vi "robot rocky222.vi"() -> ()   [LabVIEW 2021]
uses:
  <vilib>/userDefined/High Color/IMAQdx.ctl
  <vilib>/MakerHub/LINX/Private/Device/Type Defs/TCP Config.ctl
  <vilib>/vision/driver/NI_Vision_Acquisition_Software.lvlib
  <vilib>/vision/NI_Vision_Development_Module.lvlib
  <vilib>/MakerHub/LINX/LMH-LINX.lvlib
  <vilib>/MakerHub/LINX/Public/Peripherals/PWM/PWM Set Duty Cycle 1 Chan.vi
  <vilib>/MakerHub/LINX/Public/Utilities/Open TCP.vi
  <vilib>/MakerHub/LINX/Public/Peripherals/Digital/Digital Write N Chans.vi
  <vilib>/MakerHub/LINX/Private/Device/Device.lvlib
panel:
  in  "address ip":string
  in  "avance":bool
  in  "reculer":bool
  in  "Gauche":bool
  in  "droite":bool
  in  "Process Stop Button":bool
  in  "Stop":bool
  out "Image Out":T1(plugin-control)
  in  "TCP Configuration":T2
  in  "Duty Cycle (0-1)":dbl(slide) min=0.0 max=1.0 step=0.0005 scale=0.0..1.0
  in  "Motor Direction":bool[](array[boolean])
  in  "STOP":bool
  in  "Session In":T3
  in  "?":bool
  out "Acquired Frames per Second":dbl(knob) scale=0.0..100.0
  out "real time tracking":T1(plugin-control)
  in  "Color Plane":i32(ring)=1 items=["Red", "Green", "Blue", "Hue", "Saturation", "Luminance", "Value", "Intensity"]
  in  "MANUEL":bool
  in  "mode1":bool
  # "robot rocky"
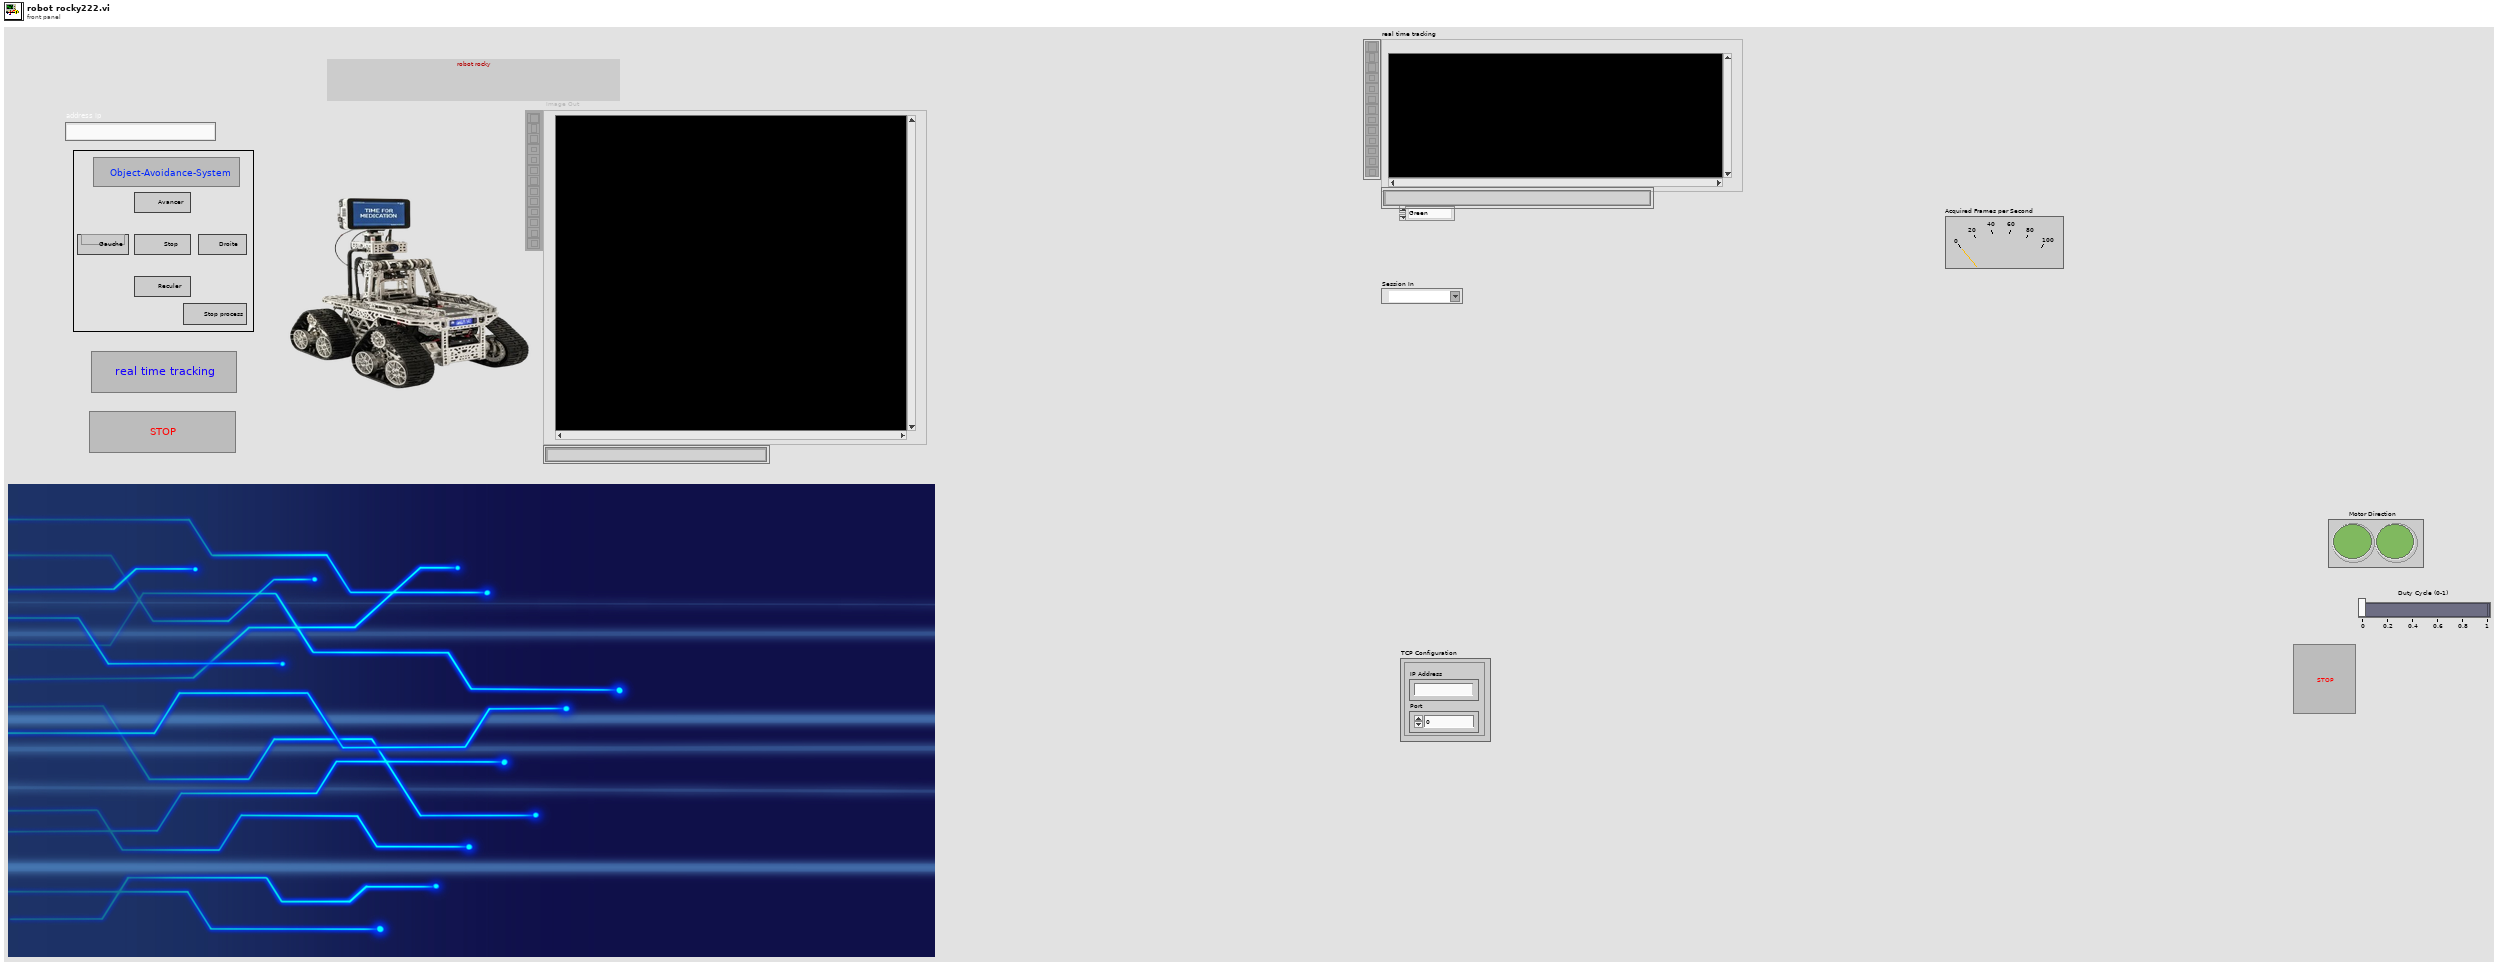
[diagram p1: front panel]
types:
  T1 = typedef "IMAQ Image.ctl" = refnum<image>
  T2 = typedef "LMH-LINX.lvlib/Device.lvlib/TCP Config.ctl" = cluster{"IP Address":string, "Port":u16}
  T3 = typedef "IMAQdx.ctl" = refnum<k21>
  T4 = typedef "Image Type" = u32
  T5 = typedef "LMH-LINX.lvlib/LINX Ref.ctl" = cluster{"IO":T6, "Interface":T7, "LINX Device Config":T8}
  T6 = typedef "LMH-LINX.lvlib/Platform.ctl" = enum16{"Remote", "Local"}
  T7 = typedef "LMH-LINX.lvlib/Interface.ctl" = enum16{"Serial", "TCP"}
  T8 = typedef "LMH-LINX.lvlib/Device.lvlib/LINX Device Config.ctl" = cluster{"Interface":T7, "COM Port":refnum<visa-resource-name>, "TCP Configuration":T2, "Device Family":u8, "Device ID":u8, "Device Name":string, "TCP Ref":refnum<k5>, "Channels":T9}
  T9 = typedef "LMH-LINX.lvlib/Channels.ctl" = cluster{"DI":u8[], "DO":u8[], "AI":u8[], "AO":u8[], "PWM":u8[], "QE":u8[], "UART":u8[], "I2C 2":u8[], "SPI":u8[], "CAN":u8[], "Servo":u8[], "AI Ref (V)":dbl, "AI Resolution (Bits)":u8, "AO Ref (V)":dbl, "AO Resolution (Bits)":u8}
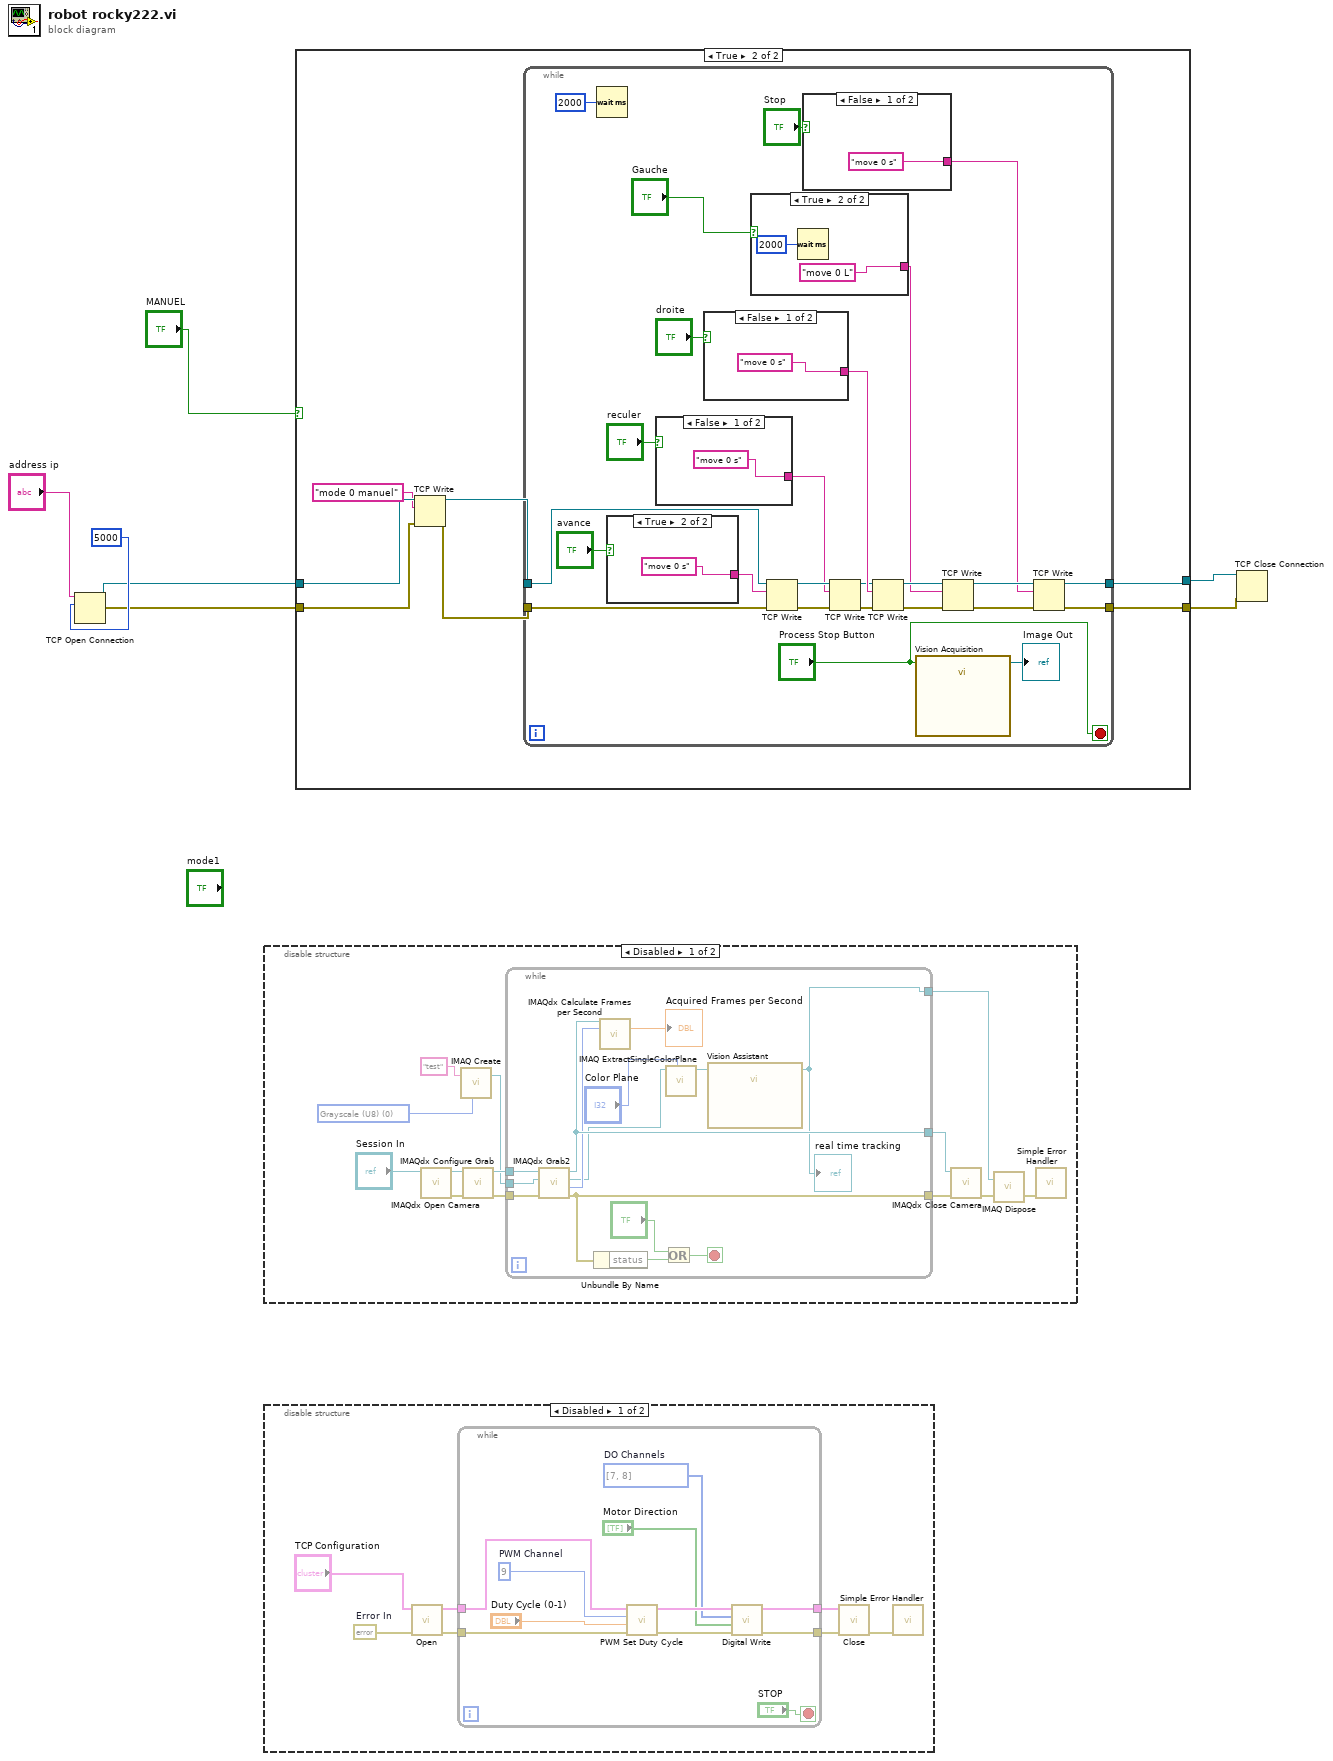
[diagram p0: block diagram]
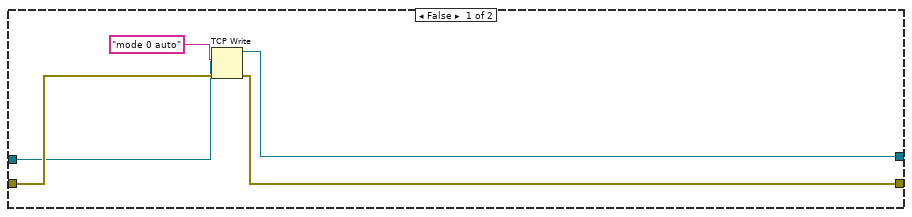
[diagram p2: hidden frame]
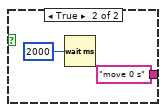
[diagram p3: hidden frame]
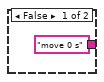
[diagram p4: hidden frame]
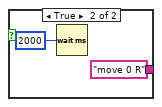
[diagram p5: hidden frame]
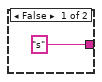
[diagram p6: hidden frame]
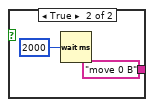
[diagram p7: hidden frame]
diagram:
  n1 = TCP Open Connection(address="address ip", remote port or service name=u16 5000) -> (connection ID=w5:refnum<k5>, error out=w4:errorcluster)  [unwired: 3 in]
  n2 = disable-structure shown="Disabled" {
    frame Disabled {
      w9 = T4 0 items=["Grayscale (U8)", "Grayscale (I16)", "Grayscale (SGL)", "Complex (CSG)", "RGB (U32)", "HSL (U32)", "RGB (U64)", "Grayscale (U16)"] ("Image Type")
      n3 = call <vilib>:"IMAQdx Open Camera.vi"("Session In"="Session In") -> ("error out"=w18:errorcluster, "Session Out"=w19:T3)  [unwired: 9 in]
      n4 = call "IMAQ Create"("Image Name"="test", "Image Type"=w9) -> ("New Image"=w8:T1)  [unwired: 3 in, 1 out]
      n5 = call <vilib>:"IMAQdx Configure Grab.vi"("error in"=w18, "Session In"=w19) -> ("error out"=w16:errorcluster, "Session Out"=w17:T3)  [unwired: 8 in]
      n6 = while {
        tunnel: w17 -> [w34]
        tunnel: w16 -> [w33]
        tunnel: [w26] -> w15
        tunnel: [w30] -> w14
        tunnel: [w21] -> w13
        tunnel: w8 -> [w28]
        stop <- w32 stop-if-true
        n7 = call <vilib>:"IMAQdx Grab2.vi"("error in"=w33, "Image In"=w28, "Session In"=w34) -> ("error out"=w30:errorcluster, "Buffer Number Out"=w25:u32, "Image Out"=w24:T1, "Session Out"=w26:T3)  [unwired: 5 in]
        n8 = Unbundle By Name(w30) -> ("status"=w29:bool)
        n9 = call <vilib>:"IMAQdx Calculate Frames per Second.vi"("Session In"=w26, "Buffer Number"=w25) -> ("Acquired Frames per Second"=→"Acquired Frames per Second":dbl)  [unwired: 7 in, 6 out]
        n10 = Or(x="?", y=w29) -> (x .or. y?=w32:bool)
        n11 = call "IMAQ ExtractSingleColorPlane"("Color Plane"="Color Plane", "Image Src"=w24) -> ("Image Dst Out"=w22:T1)  [unwired: 8 in, 1 out]
        n12 = call "Vision Assistant"("Image In"=w22) -> ("Image Out"=w21:T1)  [unwired: 25 in, 1 out]
        "real time tracking" <- w21
      }
      n13 = call <vilib>:"IMAQdx Close Camera.vi"("error in"=w14, "Session In"=w15) -> ("error out"=w12:errorcluster)  [unwired: 9 in]
      n14 = call "IMAQ Dispose"("Image"=w13, "error in (no error)"=w12) -> ("error out"=w11:errorcluster)  [unwired: 4 in]
      n15 = call <vilib>:"Simple Error Handler.vi"("error in (no error)"=w11) -> ()  [unwired: 4 in, 5 out]
    }
    frame Enabled {
    }
  }
  n16 = disable-structure shown="Disabled" {
    frame Disabled {
      w39 = errorcluster {"status"=FALSE, "code"=0, "source"=""}  # Error In
      n17 = call-poly <vilib>:"Open.vi"("Error In"=w39, "TCP Configuration"="TCP Configuration") -> ("Error Out"=w40:errorcluster, "LINX Resource"=w41:T5)  [unwired: 7 in, 1 out]
      n18 = while {
        tunnel: w41 -> [w52]
        tunnel: w40 -> [w51]
        tunnel: [w46] -> w37
        tunnel: [w45] -> w38
        stop <- "STOP" stop-if-true
        w50 = u8 9  # PWM Channel
        w42 = u8[] [7, 8]  # DO Channels
        n19 = call-poly <vilib>:"PWM Set Duty Cycle.vi"("Error In"=w51, "Duty Cycle (0-1)"="Duty Cycle (0-1)", "PWM Channel"=w50, "LINX Resource"=w52) -> ("Error Out"=w47:errorcluster, "LINX Resource"=w48:T5)  [unwired: 6 in]
        n20 = call-poly <vilib>:"Digital Write.vi"("Error In"=w47, "Values"="Motor Direction", "DO Channels"=w42, "LINX Resource"=w48) -> ("Error Out"=w46:errorcluster, "LINX Resource"=w45:T5)  [unwired: 6 in]
      }
      n21 = call <vilib>:"Close.vi"("Error In"=w37, "LINX Resource"=w38) -> ("Error Out"=w36:errorcluster)  [unwired: 9 in]
      n22 = call <vilib>:"Simple Error Handler.vi"("error in (no error)"=w36) -> ()  [unwired: 4 in, 5 out]
    }
    frame Enabled {
    }
  }
  n23 = case shown="True" "MANUEL" {
    tunnel: w5 -> [w55 w62]
    tunnel: w4 -> [w56 w59]
    tunnel: [w54 w64] -> w3
    tunnel: [w53 w63] -> w2
    frame False {
      n24 = TCP Write(connection ID=w55, data in="mode 0 auto", error in (no error)=w56) -> (connection ID out=w54:refnum<k5>, error out=w53:errorcluster)  [unwired: 1 in, 1 out]
    }
    frame True {
      n25 = TCP Write(connection ID=w62, data in="mode 0 manuel", error in (no error)=w59) -> (connection ID out=w60:refnum<k5>, error out=w58:errorcluster)  [unwired: 1 in, 1 out]
      n26 = while {
        tunnel: w60 -> [w89]
        tunnel: w58 -> [w88]
        tunnel: [w72] -> w64
        tunnel: [w71] -> w63
        stop <- "Process Stop Button" stop-if-true
        n27 = Wait (ms)(milliseconds to wait=u32 2000) -> ()  [unwired: 1 out]
        n28 = case shown="True" "avance" {
          tunnel: ["s" "move 0 s"] -> w85
          frame False {
          }
          frame True {
          }
        }
        n29 = case shown="False" "reculer" {
          tunnel: ["move 0 s" "move 0 B"] -> w84
          frame False {
          }
          frame True {
            n30 = Wait (ms)(milliseconds to wait=u32 2000) -> ()  [unwired: 1 out]
          }
        }
        n31 = case shown="False" "droite" {
          tunnel: ["move 0 s" "move 0 R"] -> w83
          frame False {
          }
          frame True {
            n32 = Wait (ms)(milliseconds to wait=u32 2000) -> ()  [unwired: 1 out]
          }
        }
        n33 = case shown="True" "Gauche" {
          tunnel: ["move 0 s" "move 0 L"] -> w78
          frame False {
          }
          frame True {
            n34 = Wait (ms)(milliseconds to wait=u32 2000) -> ()  [unwired: 1 out]
          }
        }
        n35 = TCP Write(connection ID=w89, data in=w85, error in (no error)=w88) -> (connection ID out=w87:refnum<k5>, error out=w86:errorcluster)  [unwired: 1 in, 1 out]
        n36 = case shown="False" "Stop" {
          tunnel: ["move 0 s" ("write buffer") "move 0 s"] -> w70
          frame False {
          }
          frame True {
            n37 = Wait (ms)(milliseconds to wait=u32 2000) -> ()  [unwired: 1 out]
          }
        }
        n38 = TCP Write(connection ID=w87, data in=w84, error in (no error)=w86) -> (connection ID out=w82:refnum<k5>, error out=w81:errorcluster)  [unwired: 1 in, 1 out]
        n39 = TCP Write(connection ID=w82, data in=w83, error in (no error)=w81) -> (connection ID out=w79:refnum<k5>, error out=w80:errorcluster)  [unwired: 1 in, 1 out]
        n40 = call "Vision Acquisition"("Stop (F)"="Process Stop Button") -> ("Image Out"=→"Image Out":T1)  [unwired: 24 in, 2 out]
        n41 = TCP Write(connection ID=w79, data in=w78, error in (no error)=w80) -> (connection ID out=w77:refnum<k5>, error out=w76:errorcluster)  [unwired: 1 in, 1 out]
        n42 = TCP Write(connection ID=w77, data in=w70, error in (no error)=w76) -> (connection ID out=w72:refnum<k5>, error out=w71:errorcluster)  [unwired: 1 in, 1 out]
      }
    }
  }
  n43 = TCP Close Connection(connection ID=w3, error in (no error)=w2) -> ()  [unwired: 1 in, 2 out]
